vi "Terminal Configuration to String.vi"(11 "terminal configuration":T1 items=[""=-1, "differential"=10106, "pseudodifferential"=12529]) -> (3 "f":string)   [LabVIEW 2019, in "Instrument.Lockin.lvlib" / "Instrument.Lockin.lvclass"]
uses:
  Instrument.Lockin.lvclass
  Instrument.DAQ/Typedefs/DAQ.TerminalConfiguration--ring.ctl
  Instrument.DAQ/Instrument.DAQ.lvclass
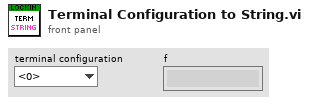
[diagram p1: front panel]
types:
  T1 = typedef "Instrument.Lockin.lvlib/Instrument.DAQ.lvclass/DAQ.TerminalConfiguration--ring.ctl" = i32
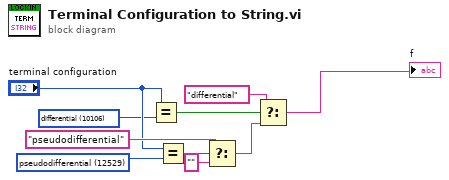
[diagram p0: block diagram]
diagram:
  w5 = T1 12529 items=[""=-1, "differential"=10106, "pseudodifferential"=12529] ("terminal configuration")
  w1 = T1 10106 items=[""=-1, "differential"=10106, "pseudodifferential"=12529] ("terminal configuration")
  n1 = Equal?(x="terminal configuration", y=w1) -> (x = y?=w2:bool)
  n2 = Equal?(x="terminal configuration", y=w5) -> (x = y?=w7:bool)
  n3 = Select(t="pseudodifferential", s=w7, f="") -> (s? t:f=w8:string)
  n4 = Select(t="differential", s=w2, f=w8) -> (s? t:f=→"f":string)
